vi "Library Paths.vi"(8 "error in (no error)":errorcluster, 11 "Base Dir in":path) -> (0 "error out":errorcluster, 1 "Project Libraries (.lvlib)":path[](array[path]), 2 "Packed Libraries (.lvlibp)":path[](array[path]), 3 "Base Dir out":path)   [LabVIEW 2018, in "Shared.lvlib"]
uses:
  Shared.lvlib
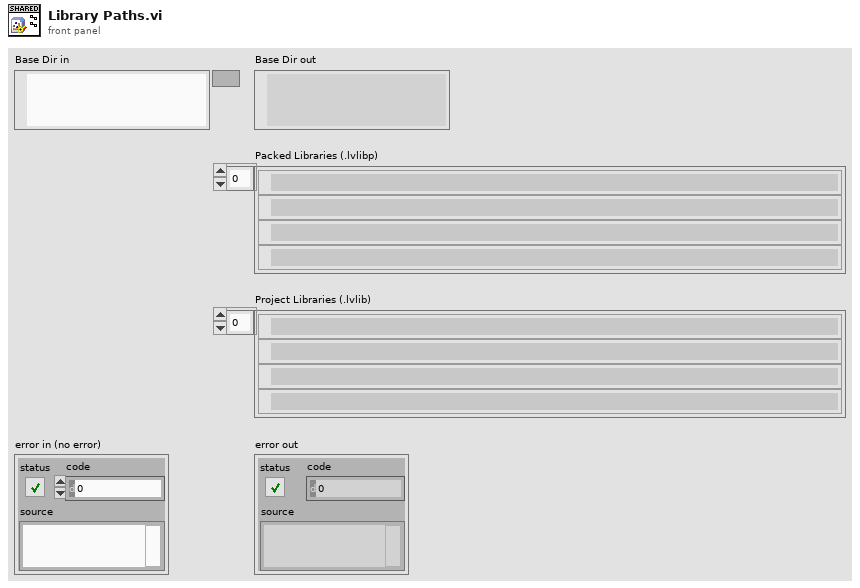
[diagram p1: front panel]
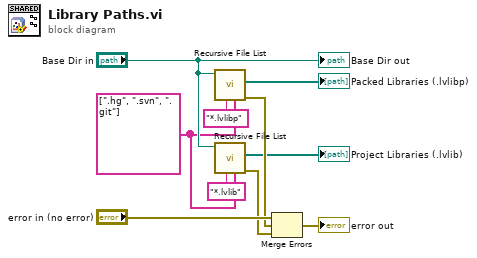
[diagram p0: block diagram]
diagram:
  w6 = string[] [".hg", ".svn", ".git"] ("Folders to Exclude")
  n1 = call <vilib>:"Recursive File List.vi"("Folders to Exclude"=w6, "pattern"="*.lvlibp", "Folder Path"="Base Dir in") -> ("error out"=w3:errorcluster, "All Files in Dir"=→"Packed Libraries (.lvlibp)":path[])  [unwired: 4 in, 3 out]
  n2 = call <vilib>:"Recursive File List.vi"("Folders to Exclude"=w6, "pattern"="*.lvlib", "Folder Path"="Base Dir in") -> ("error out"=w2:errorcluster, "All Files in Dir"=→"Project Libraries (.lvlib)":path[])  [unwired: 4 in, 3 out]
  n3 = Merge Errors("error in (no error)", w3, w2) -> (→"error out":errorcluster)
  "Base Dir out" <- "Base Dir in"
